vi "Read Multiple Points.vi"(8 "error in (no error)":errorcluster, 11 "Simulated DMM in":refnum<class "Simulated DMM.lvclass">) -> (0 "error out":errorcluster, 2 "Waveform":waveform(dbl), 3 "Simulated DMM out":refnum<class "Simulated DMM.lvclass">)   [LabVIEW 2017, in "Simulated DMM.lvclass"]
uses:
  Simulated DMM.lvclass
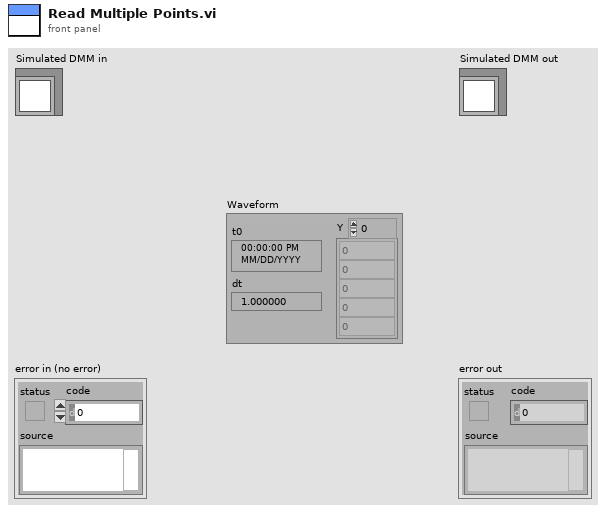
[diagram p1: front panel]
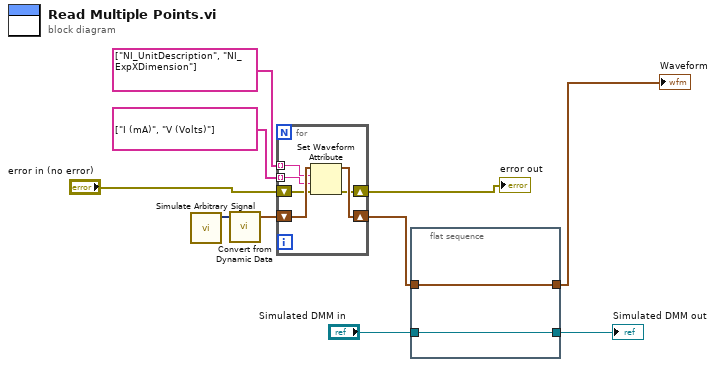
[diagram p0: block diagram]
diagram:
  n1 = call "Simulate Arbitrary Signal"() -> ("Signal"=w6:dynamicdata)  [unwired: 9 in, 2 out]
  n2 = call "Convert from Dynamic Data"("Dynamic Data Type"=w6) -> ("Waveform"=w7:waveform(dbl))  [unwired: 3 in]
  n3 = for {
    shift-right: [w15] -> w10
    shift-left: w7 -> [w16]
    tunnel: string[] ["NI_UnitDescription", "NI_ExpXDimension"] -> [w14] mode=indexing
    tunnel: string[] ["I (mA)", "V (Volts)"] -> [w13] mode=indexing
    shift-right: [w11] -> w2
    shift-left: "error in (no error)" -> [w12]
    n4 = Set Waveform Attribute(4:w12, 5:w13, 6:w14, 7:w16) -> (0:w11:errorcluster, 3:w15:waveform(dbl))  [unwired: 1 out]
  }
  "error out" <- w2
  n5 = flat-sequence {
    tunnel: w10 -> [w18]
    tunnel: [w18] -> w5
    tunnel: [w17] -> w3
    tunnel: "Simulated DMM in" -> [w17]
    frame #0 {
    }
  }
  "Simulated DMM out" <- w3
  "Waveform" <- w5
